vi "Scene3_STLfile_(SubVI).vi"() -> (0 "error out":errorcluster, 2 "New Object Out":refnum<vi>, 3 "SceneObject out":refnum<vi>)   [LabVIEW 2013]
uses:
  <vilib>/picture/3D Picture Control/NI_3D Picture Control.lvlib
  <vilib>/picture/3D Picture Control/Object/Create Object (drawable).vi
  <vilib>/picture/3D Picture Control/Object/Add Object (reference).vi
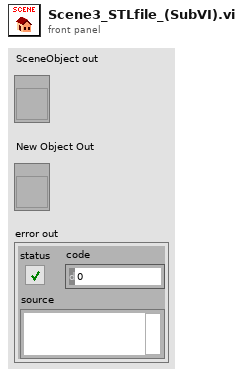
[diagram p1: front panel]
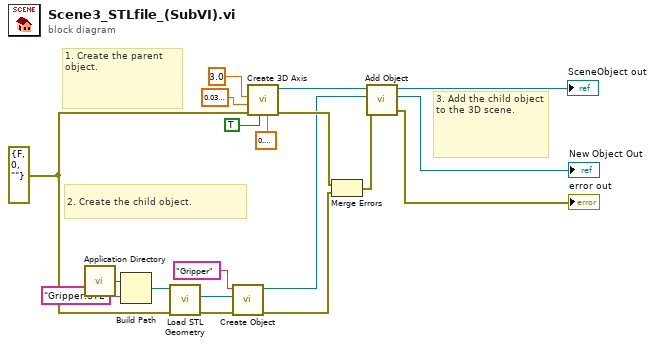
[diagram p0: block diagram]
diagram:
  w5 = errorcluster {"status"=FALSE, "code"=0, "source"=""} ("error in (no error)")
  # "2. Create the child object."
  # "3. Add the child object to the 3D scene."
  # "1. Create the parent object."
  n1 = call <vilib>:"Application Directory.vi"() -> ("Application Directory"=w3:path)
  n2 = Build Path(base path=w3, name or relative path="Gripper.STL") -> (appended path=w1:path)
  n3 = call <vilib>:"Load STL Geometry.vi"("error in (no error)"=w5, "Model File"=w1) -> ("error out"=w4:errorcluster, "New Mesh Refnum"=w6:refnum<vi>)  [unwired: 8 in]
  n4 = call-poly <vilib>:"Create Object.vi"("error in (no error)"=w4, "Geometry"=w6, "Name"="Gripper") -> ("error out"=w7:errorcluster, "Scene:New Object"=w8:refnum<vi>)  [unwired: 7 in]
  n5 = call <vilib>:"Create 3D Axis.vi"("Character Size"=sgl 0.4, "Axis label?"=TRUE, "error in (no error)"=w5, "Radius"=sgl 0.04, "Length"=sgl 3.0) -> ("error out"=w11:errorcluster, "New Object Refnum"=w14:refnum<vi>)  [unwired: 5 in]
  n6 = Merge Errors(w11, w7) -> (w10:errorcluster)
  n7 = call-poly <vilib>:"Add Object.vi"("error in (no error)"=w10, "New Object In"=w8, "Scene Object In"=w14) -> ("error out"=→"error out":errorcluster, "New Object Out"=→"New Object Out":refnum<vi>, "Scene Object Out"=→"SceneObject out":refnum<vi>)  [unwired: 6 in]
